vi "CPP-ZeroMaintenance.vi"(1 "Previous Scan Value":dbl, 2 "Ch Description":T2={"Ch Name"="Tunnel3:Pressures:", "Type"="", "Function"=enum."Analogue Input", "Ch State"=enum."On", "Calibration type"=enum."Raw", "A"=30.0, "B"=10.0, "C"=0.0, "D"=0.0, "Comments"="", "Address"={"Main"=0, "Ch."=0, "Sub"=0, "Port Name"=""}, "String"="", "Duty"=65535} {"Duty" format="%.0b"; "D" format="%#_5g"; "C" format="%#_5g"; "B" format="%#_5g"; "A" format="%#_5g"}) -> (0 "Time Elapsed since zero (min)":dbl format="%#.2f")   [LabVIEW 2015]
doc: "This VI performs the Auto Zeroing routine. All of the information for a given Rig should be included in the Channel Description for this to work correctly. The Channel name is not terribly important, but the assumed convention is < Rig Name >:Pressures:\n\nA := Seconds to Monitor is the interval used to determine whether the tunnel has been off long enough\nB := Seconds to Average is the averaging interval for recording zeroes\nC := timestamp of most recent Zero\nD := timestamp of previous Zero\n\nThe String element should be a semi-colon-separated array of ADAM Chs. The first Ch in the array should be the Listener Ch which is compared with the Threshold to determine if the tunnel is OFF. The remaining array of ADAM Chs should be all of the Pressure Chs that are to be auto-zeroed."
uses:
  ADAM Client/Sub VIs/ADAM Controls/Ch_description_ADAM.ctl
  ADAM Client/Sub VIs/ADAM Controls/Module_type_ADAM.ctl
  ADAM Client/Sub VIs/ADAM Controls/Function_ADAM.ctl
  ADAM Client/Sub VIs/ADAM Controls/Channel_State.ctl
  ADAM Client/Sub VIs/ADAM Controls/Calib_type_ADAM.ctl
  ADAM Client/Sub VIs/ADAM Controls/Address.ctl
panel:
  in  "Tab Control":T1(tab)
  out "Listener Threshold":dbl
  out "Fresh Data Available?":bool
  out "Do Zeroes?":bool
  out "Below Threshold?":bool
  out "Listening Ch":string[](array[string])
  out "Pressure Chs":string[](array[string])
  out "Listening Value":dbl=0.2694398123338766
  out "current time":timestamp=timestamp(3521053420.076362 s since 1904-01-01)
  out "Current Time (sec)":dbl=3521053420.076362 format="%#.0f"
  out "LastZeroedSS":dbl=3521053410.165856 format="%#.0f"
  in  "Throwback (s)":dbl=10.0 format="%#_13g"
  # "This VI performs the Auto Zeroing routine. All of the information for a given Rig should be included in the Channel Description for this to work correctly. The Channel name is not terribly important, but the assumed convention is < Rig Name >:Pressures:\n\nA := Seconds to Monitor is the interval used to determine whether the tunnel has been off long enough\nB := Seconds to Average is the averaging interval for recording zeroes\nC := timestamp of most recent Zero\nD := threshold to consider zeroing\n\nThe String element should be a semi-colon-separated array of ADAM Chs. The first Ch in the array should be the Listener Ch which is compared with the Threshold to determine if the tunnel is ON. The remaining array of ADAM Chs should be all of the Pressure Chs that are to be auto-zeroed."
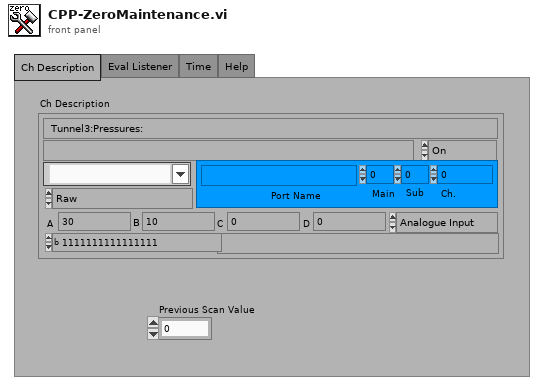
[diagram p1: front panel]
types:
  T1 = enum32{"Ch Description", "Eval Listener", "Time", "Help"}
  T2 = typedef "Ch_description_ADAM.ctl" = cluster{"Ch Name":string, "Type":T3, "Function":T4, "Ch State":T5, "Calibration type":T6, "A":dbl, "B":dbl, "C":dbl, "D":dbl, "Comments":string, "Address":T7, "String":string, "Duty":u16}
  T3 = typedef "Module_type_ADAM.ctl" = string
  T4 = typedef "Function_ADAM.ctl" = enum16{"Analogue Input", "Digital Input", "Event counter", "Event rate", "Analogue Output", "Digital Output", "Relay Output"}
  T5 = typedef "Channel_State.ctl" = enum16{"On", "Off", "Always On", "Always Off"}
  T6 = typedef "Calib_type_ADAM.ctl" = enum16{"Raw", "Bx + A", "Cx^2 + Bx + A", "Dx^3 + Cx^2 + Bx + A", "In Band", "Hi-Tec Q", "Hi-Tec M_dot", "Text"}
  T7 = typedef "Address.ctl" = cluster{"Main":i32, "Ch.":i32, "Sub":i32, "Port Name":string}
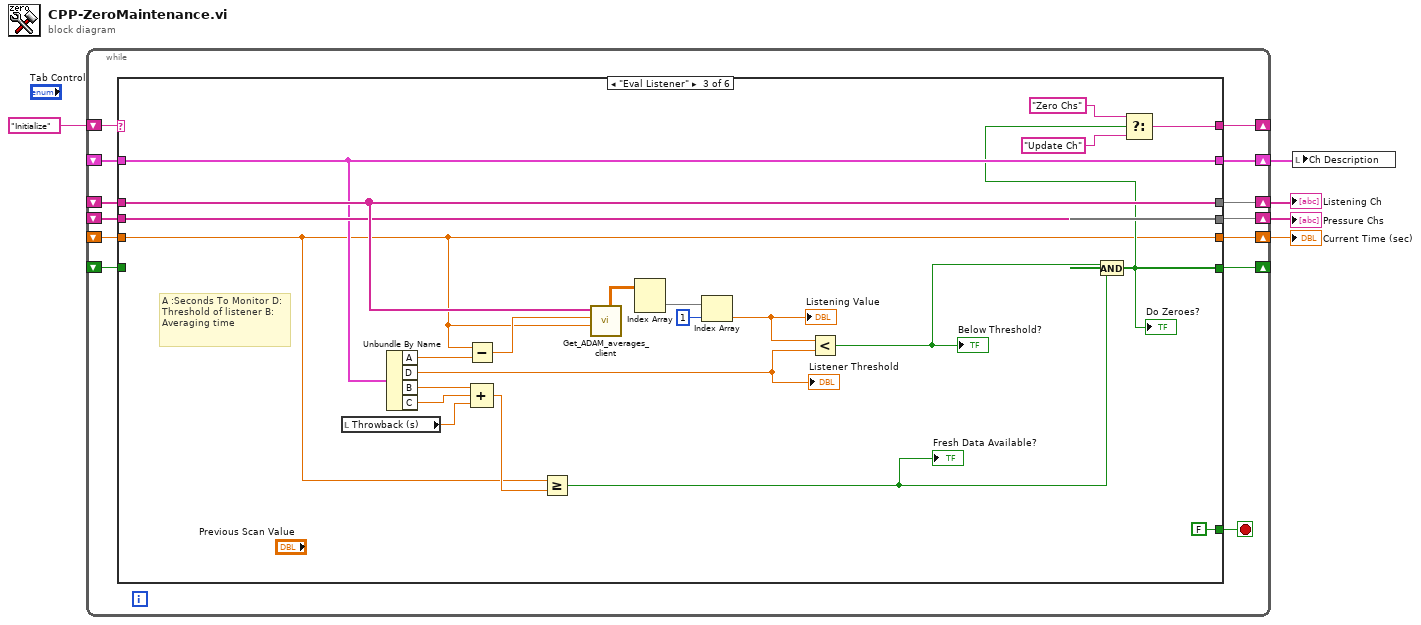
[diagram p0: block diagram]
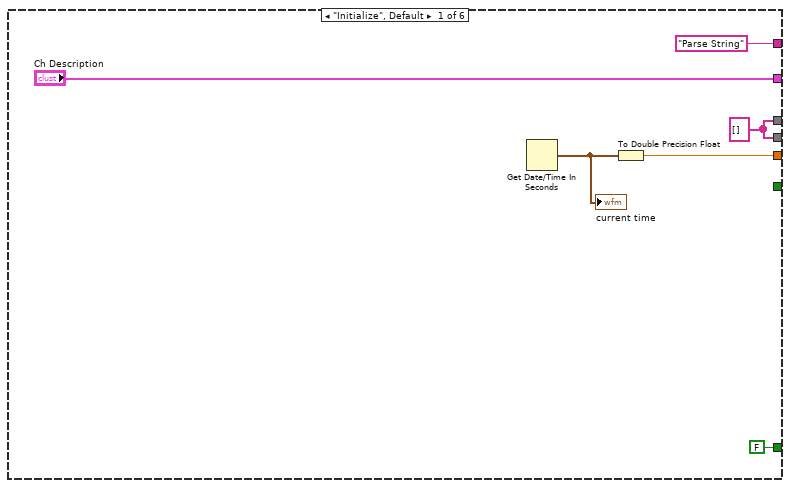
[diagram p2: hidden frame]
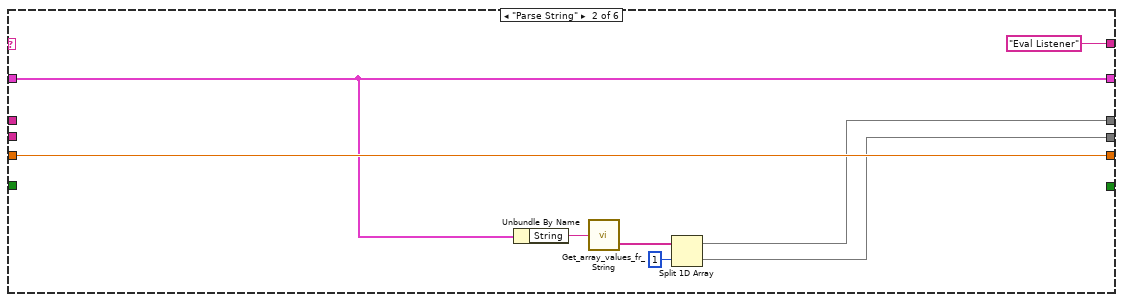
[diagram p3: hidden frame]
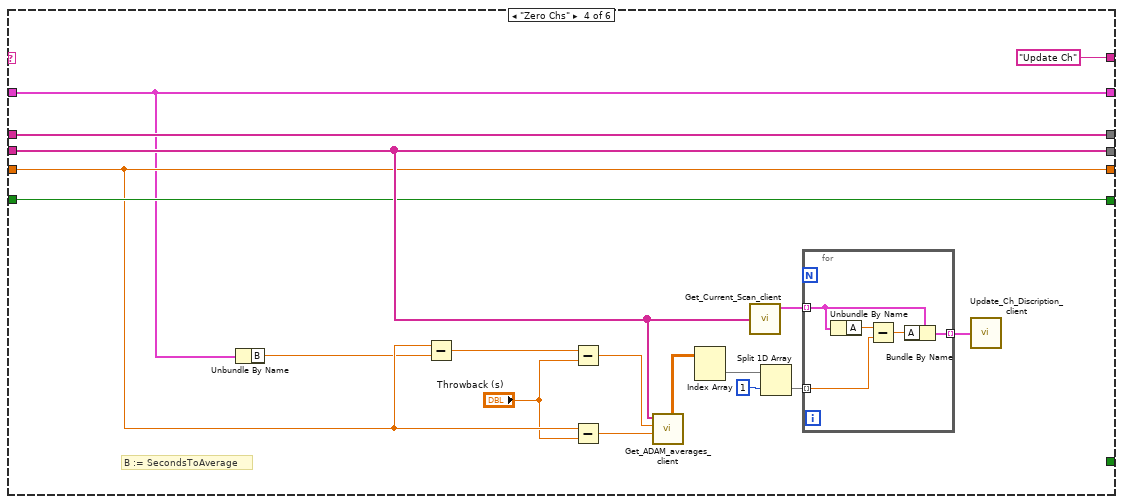
[diagram p4: hidden frame]
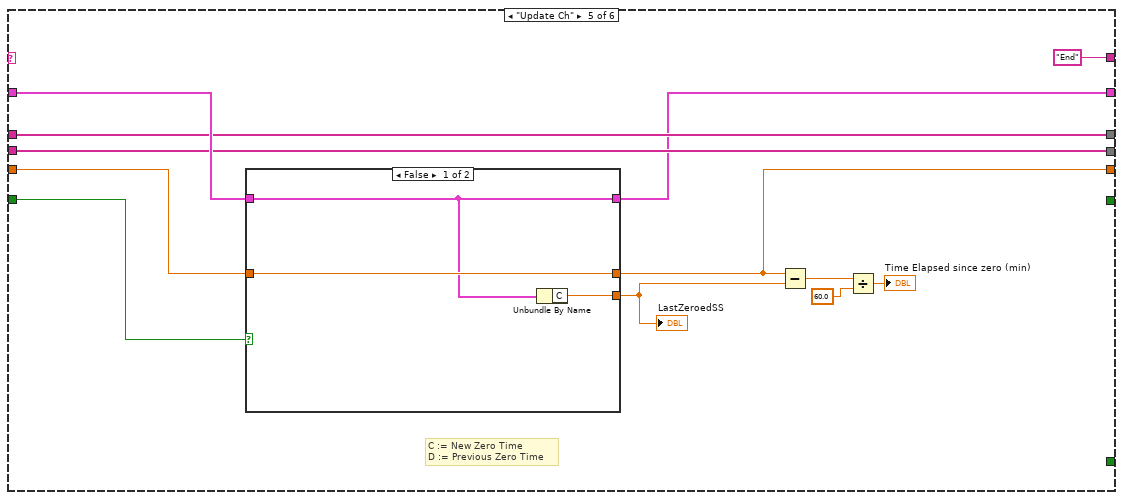
[diagram p5: hidden frame]
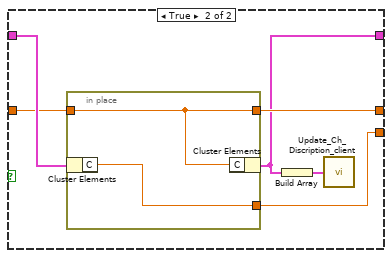
[diagram p6: hidden frame]
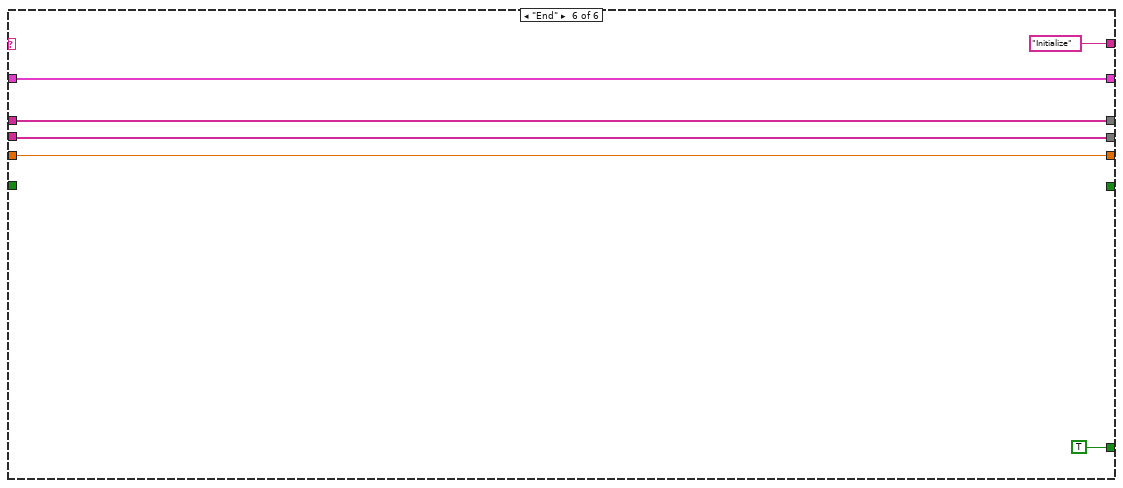
[diagram p7: hidden frame]
diagram:
  n1 = while {
    shift-right: [w17] -> _
    shift-left: "Initialize" -> [w18]
    shift-right: [w15] -> w1
    shift-left: _ -> [w16]
    shift-right: [w14] -> w3
    shift-left: _ -> [w13]
    shift-right: [w12] -> w2
    shift-left: _ -> [w11]
    shift-right: [w10] -> w4
    shift-left: _ -> [w8]
    shift-right: [w7] -> _
    shift-left: _ -> [w6]
    stop <- w9 stop-if-true
    n2 = case shown="\"Eval Listener\"" w18 {
      tunnel: ["Parse String" "Eval Listener" w44 "Update Ch" "End" "Initialize"] -> w17
      tunnel: w16 -> [_ w29 w49 w66 w88 w104]
      tunnel: ["Ch Description" w29 w49 w66 w78 w104] -> w15
      tunnel: [w21 w26 w51 w70 w80 w102] -> w14
      tunnel: w13 -> [_ _ w51 w70 w80 w102]
      tunnel: [w21 w25 w50 w71 w79 w101] -> w12
      tunnel: w11 -> [_ _ w50 w71 w79 w101]
      tunnel: [w23 w30 w35 w67 w82 w100] -> w10
      tunnel: [FALSE _ FALSE _ _ TRUE] -> w9
      tunnel: w8 -> [_ w30 w35 w67 w86 w100]
      tunnel: [_ _ w38 w69 _ _] -> w7
      tunnel: w6 -> [_ _ _ w69 w87 _]
      frame "Initialize", Default {
        w21 = string[] []
        n3 = Get Date/Time In Seconds() -> (seconds since 1Jan1904=w24:timestamp)
        "current time" <- w24
        n4 = To Double Precision Float(number=w24) -> (double precision float=w23:dbl)
      }
      frame "Parse String" {
        n5 = Unbundle By Name(w29) -> ("String"=w31:string)
        n6 = call "Get_array_values_fr_String.vi"("String Value"=w31) -> ("String array"=w28:string[])  [unwired: 1 out]
        n7 = Split 1D Array(array=w28, index=1) -> (first subarray=w26:string[], second subarray=w25:string[])
      }
      frame "Eval Listener" {
        # "A :Seconds To Monitor D: Threshold of listener B: Averaging time"
        n8 = local read "Throwback (s)"() -> (w33:dbl)
        n9 = Unbundle By Name(w49) -> ("A"=w48:dbl, "D"=w36:dbl, "B"=w37:dbl, "C"=w34:dbl)
        "Listener Threshold" <- w36
        n10 = Subtract(x=w35, y=w48) -> (x-y=w52:dbl)
        n11 = Compound Arithmetic op=ADD(w37, w34, w33) -> (w40:dbl)
        n12 = Greater Or Equal?(x=w35, y=w40) -> (x >= y?=w41:bool)
        "Fresh Data Available?" <- w41
        n13 = call "Get_ADAM_averages_client.vi"("End time"=w35, "Start time"=w52, "ADAM Ch Names"=w51) -> ("DBL values"=w54:dbl[][])  [unwired: 4 in, 4 out]
        n14 = Index Array(array=w54) -> (element=w53:dbl[])  [unwired: 2 in]
        n15 = Index Array(array=w53, index=1) -> (element=w39:dbl)
        "Listening Value" <- w39
        n16 = Less?(x=w39, y=w36) -> (x < y?=w42:bool)
        "Below Threshold?" <- w42
        n17 = And(x=w42, y=w41) -> (x .and. y?=w38:bool)
        "Do Zeroes?" <- w38
        n18 = Select(t="Zero Chs", s=w38, f="Update Ch") -> (s? t:f=w44:string)
      }
      frame "Zero Chs" {
        # "B := SecondsToAverage"
        n19 = Unbundle By Name(w66) -> ("B"=w65:dbl)
        n20 = Subtract(x=w67, y=w65) -> (x-y=w61:dbl)
        n21 = Subtract(x=w61, y="Throwback (s)") -> (x-y=w62:dbl)
        n22 = Subtract(x=w67, y="Throwback (s)") -> (x-y=w63:dbl)
        n23 = call "Get_ADAM_averages_client.vi"("End time"=w63, "Start time"=w62, "ADAM Ch Names"=w71) -> ("DBL values"=w56:dbl[][])  [unwired: 4 in, 4 out]
        n24 = Index Array(array=w56) -> (element=w57:dbl[])  [unwired: 2 in]
        n25 = call "Get_Current_Scan_client.vi"("ADAM Ch Names"=w71) -> ("Ch Description Array"=w55:T2[])  [unwired: 3 out]
        n26 = Split 1D Array(array=w57, index=1) -> (second subarray=w58:dbl[])  [unwired: 1 out]
        n27 = for {
          tunnel: w55 -> [w74] mode=indexing
          tunnel: w58 -> [w75] mode=indexing
          tunnel: [w72] -> w60 mode=indexing
          n28 = Unbundle By Name(w74) -> ("A"=w76:dbl)
          n29 = Subtract(x=w76, y=w75) -> (x-y=w73:dbl)
          n30 = Bundle By Name(cluster=w74, "A"=w73) -> (w72:T2)
        }
        n31 = call "Update_Ch_Discription_client.vi"("Channels to update In"=w60) -> ()  [unwired: 1 out]
      }
      frame "Update Ch" {
        # "C := New Zero Time\nD := Previous Zero Time"
        n32 = case shown="False" w87 {
          tunnel: w88 -> [w90 w97]
          tunnel: w86 -> [w91 w96]
          tunnel: [w91 w93] -> w82
          tunnel: [w89 w94] -> w77
          tunnel: [w90 w92] -> w78
          frame False {
            n33 = Unbundle By Name(w90) -> ("C"=w89:dbl)
          }
          frame True {
            n34 = in-place {
              in-place-border: w96 -> [w99]
              in-place-border: [w99] -> w93
              in-place-border: [w98] -> w94
              n35 = in-place-cluster #1(w97) -> ("C"=w98:dbl)
              n36 = in-place-cluster #1("C"=w99) -> (w92:T2)
            }
            n37 = Build Array(w92) -> (w95:T2[])
            n38 = call "Update_Ch_Discription_client.vi"("Channels to update In"=w95) -> ()  [unwired: 1 out]
          }
        }
        "LastZeroedSS" <- w77
        n39 = Subtract(x=w82, y=w77) -> (x-y=w83:dbl)
        n40 = Divide(x=w83, y=60.0) -> (x/y=→"Time Elapsed since zero (min)":dbl)
      }
      frame "End" {
      }
    }
  }
  "Current Time (sec)" <- w4
  "Listening Ch" <- w3
  "Pressure Chs" <- w2
  n41 = local write "Ch Description"(w1) -> ()
